vi "Meas Asynchronous Start.vi"(8 "error in":errorcluster, 10 "parameter in":variant, 11 "Static VI reference in (empty)":refnum<vi>) -> (0 "error out":errorcluster, 3 "async VI reference out":refnum<vi>)   [LabVIEW 2018]
doc: "Starts VI asynchronously, i.e. it will run it as another thread/process on backgroun in parallel with calling VI. This VI will return immediately. Exit state of the executed VI must be checked periodically either using standard 'Wait On Asynchronous Call' or by more comfortable 'Meas Asynchronous Wait'. In both cases the VI checks the exit status and if the VI just exited it will return its output variables. Note that output variables are returned only once after exit, then system destroys reference and deallocates VI's data.\nNote that it is not bad idea to check status of the asycnhronous VI before exitting programm and if it is still running then somehow force it to terminate so nothing stays in memory on background."
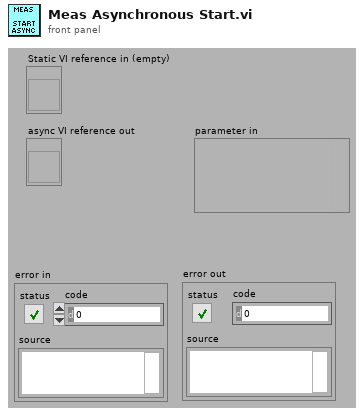
[diagram p1: front panel]
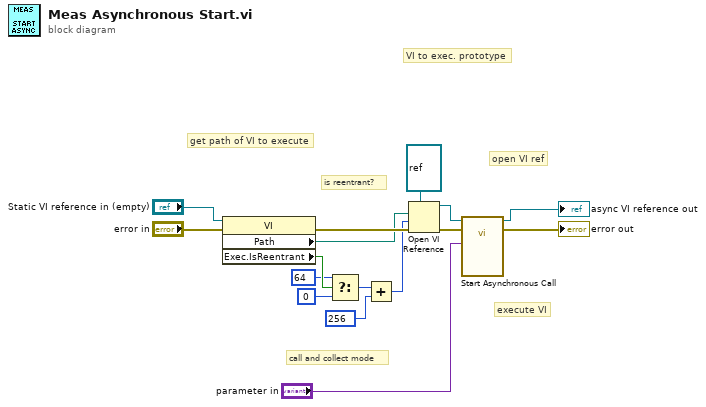
[diagram p0: block diagram]
diagram:
  # "execute VI"
  # "open VI ref"
  # "VI to exec. prototype"
  # "get path of VI to execute"
  # "is reentrant?"
  # "call and collect mode"
  n1 = property class="VI"(reference="Static VI reference in (empty)", error in="error in") -> (error out=w14:errorcluster, "Path"=w13:path, "Exec.IsReentrant"=w9:bool)  [unwired: 1 out]
  n2 = Select(t=64 ("options"), s=w9, f=0 ("options")) -> (s? t:f=w8:i32)
  n3 = Add(x=w8, y=256 ("options")) -> (x+y=w4:i32)
  n4 = Open VI Reference(type specifier VI Refnum (for type only)=refnum<vi> refnum, vi path=w13, options=w4, error in (no error)=w14) -> (vi reference=w10:refnum<vi>, error out=w11:errorcluster)  [unwired: 2 in]
  n5 = call-by-ref "Start Asynchronous Call"(reference=w10, error in=w11, "session in"="parameter in") -> (reference out=→"async VI reference out":refnum<vi>, error out=→"error out":errorcluster)  [unwired: 9 in, 2 out]
